vi "HiTechnic IRSeeker Sensor_AC all.vi"(0 "AC Mode":u8(ring) items=["1200 Hz", "600 Hz"], 2 "NXT":T4={"error"={"status"=FALSE, "code"=0, "source"=""}, "address"="", "NXT #"=-1, "Show Error"=TRUE, "Connection"=4} {"Connection" items=["USB", "Bluetooth", "USB then Bluetooth", "Last Connection", "Preference"]}, 3 "Port/MUX":T2 {"Port" items=["Port 1", "Port 2", "Port 3", "Port 4"]; "MUX Port" items=["No MUX", "MUX 1", "MUX 2", "MUX 3", "MUX 4"]}) -> (1 "All Info":T1, 4 "NXT":T4={"error"={"status"=FALSE, "code"=0, "source"=""}, "address"="", "NXT #"=-1, "Show Error"=TRUE, "Connection"=4} {"Connection" items=["USB", "Bluetooth", "USB then Bluetooth", "Last Connection", "Preference"]})   [LabVIEW 2009]
doc: "Reads the HiTechnic IRSeeker V2 Sensor in AC mode connected to the specified port and outputs a cluster containing the direction value as well an array of signal strengths from the five internal IR sensor elements. The direction value is in the range of 0 to 9 with 0 representing no IR detected; 1 to 9 represents a direction in a CW semi-circle around the sensor of which 5 indicates the IR source is straight ahead. In AC mode the sensor concentrates on a pulsating signal of either 600Hz or 1200Hz depending on the AC Mode setting.\n\n<B>Inputs\nNXT </B> connects to NXT terminal of previous VI to establish the flow of the program.\n<B>Port/MUX </B> is the port used for the sensor. This is a cluster that consists of the NXT port as well as the HiTechnic Sensor Multiplexer (MUX) port. If the MUX is not used, then set this field to <B>No MUX</B>.\n<B>AC Mode </B> can be set to either 600 Hz or 1200 Hz (default).\n\n<B>Outputs\nNXT </B> wires to NXT terminal of next VI to establish the flow of the program.\n<B>All Info </B> is a cluster containing the direction value as well as a 5 element array of signal strengths."
uses:
  <vilib>/NXT/Subs/LVHSConnector.ctl
  <vilib>/NXT/HiTechnic/subVIs/HiTechnic Port.ctl
  <vilib>/NXT/Block Support/NXT_InputPort.ctl
panel:
  in  "Previous Mode":u8[](array[ring])=[0, 0, 0, 0] items=["1200 Hz", "600 Hz"]
  # "HiTechnic IRSeeker Sensor VI\n\nThis VI reads the HiTechnic IRSeeker Sensor and \nreturns the current heading.\n\nFor more information go to www.hitechnic.com\nor email support@hitechnic.com\n(c) 2007 - 2009 HiTechnic"
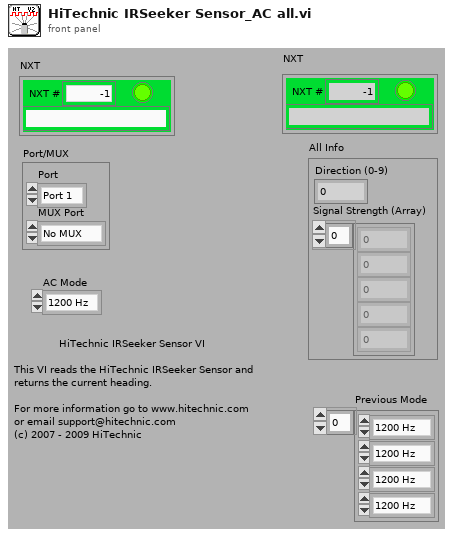
[diagram p1: front panel]
types:
  T1 = cluster{"Direction (0-9)":u8, "Signal Strength (Array)":u8[]}
  T2 = typedef "HiTechnic Port.ctl" = cluster{"Port":T3, "MUX Port":u8}
  T3 = typedef "NXT_InputPort.ctl" = u8
  T4 = typedef "LVHSConnector.ctl" = cluster{"error":errorcluster, "address":string, "NXT #":i32, "Show Error":bool, "Connection":u16}
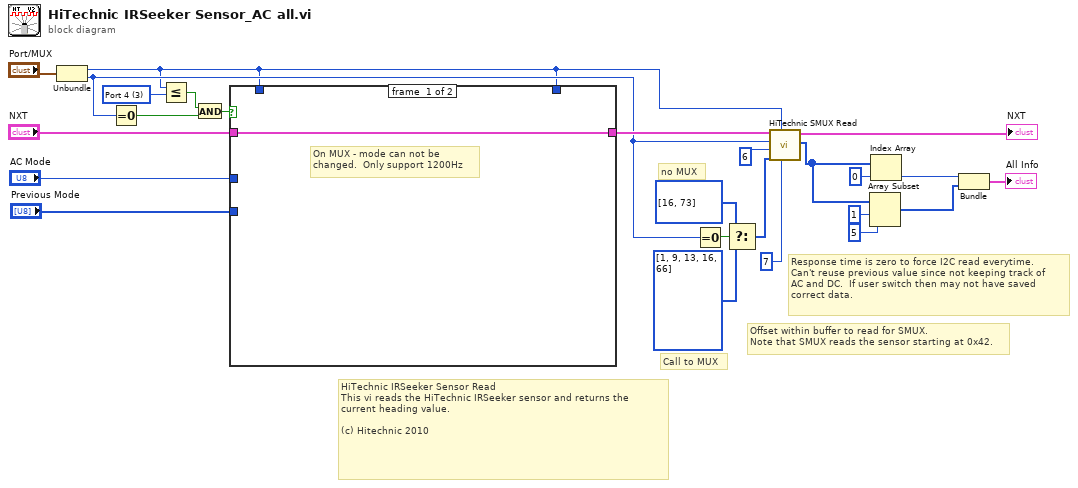
[diagram p0: block diagram]
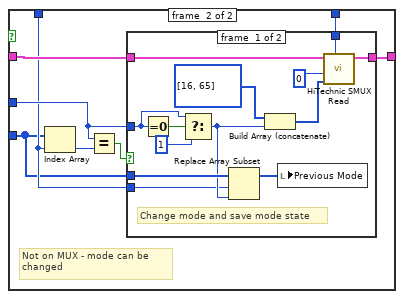
[diagram p2: hidden frame]
diagram:
  w4 = T3 3 items=["Port 1", "Port 2", "Port 3", "Port 4"] ("y")
  # "Response time is zero to force I2C read everytime.\nCan't reuse previous value since not keeping track of\nAC and DC.  If user switch then may not have saved \ncorrect data."
  # "Offset within buffer to read for SMUX.  \nNote that SMUX reads the sensor starting at 0x42."
  # "no MUX"
  # "Call to MUX"
  # "HiTechnic IRSeeker Sensor Read\nThis vi reads the HiTechnic IRSeeker sensor and returns the\ncurrent heading value.  \n\n(c) Hitechnic 2010"
  n1 = Unbundle("Port/MUX") -> ("Port"=w5:T3, "MUX Port"=w6:u8)
  n2 = Equal To 0?(x=w6) -> (x = 0?=w2:bool)
  n3 = Less Or Equal?(x=w5, y=w4) -> (x <= y?=w3:bool)
  n4 = And(x=w3, y=w2) -> (x .and. y?=w1:bool)
  n5 = case shown="True" w1 {
    tunnel: "NXT" -> [w26 w33]
    tunnel: [w26 w32] -> w9
    tunnel: "Previous Mode" -> [_ w28]
    tunnel: w5 -> [_ w30]
    tunnel: "AC Mode" -> [_ w31]
    tunnel: w5 -> [_ w29]
    frame #0 {
      # "On MUX - mode can not be\nchanged.  Only support 1200Hz"
    }
    frame #1 {
      # "Not on MUX - mode can be \nchanged"
      n6 = Index Array(array=w28, index=w30) -> (element=w34:u8)
      n7 = Equal?(x=w31, y=w34) -> (x = y?=w27:bool)
      n8 = case shown="True" w27 {
        tunnel: w33 -> [w46 w48]
        tunnel: [w45 w48] -> w32
        tunnel: w31 -> [w43 _]
        tunnel: w28 -> [w39 _]
        tunnel: w30 -> [w37 _]
        tunnel: w29 -> [w35 _]
        frame #0 {
          # "Change mode and save mode state"
          n9 = Equal To 0?(x=w43) -> (x = 0?=w44:bool)
          n10 = Select(t=w43, s=w44, f=u8 1) -> (s? t:f=w38:u8)
          n11 = Replace Array Subset(array=w39, new element=w38, index=w37) -> (w36:u8[])
          n12 = Build Array (concatenate)(u8[] [16, 65] ("Buffer"), w38) -> (w40:u8[])
          n13 = local write "Previous Mode"(w36) -> ()
          n14 = call <vilib>:"HiTechnic SMUX Read.vi"("Port"=w35, "Parameters"=w40, "Read Length"=0, "NXT"=w46) -> ("NXT"=w45:T4)  [unwired: 6 in, 1 out]
        }
        frame #1 {
          # "Mode not changed."
        }
      }
    }
  }
  n15 = Equal To 0?(x=w6) -> (x = 0?=w22:bool)
  n16 = Select(t=u8[] [16, 73] ("Buffer"), s=w22, f=u8[] [1, 9, 13, 16, 66]) -> (s? t:f=w25:u8[])
  n17 = call <vilib>:"HiTechnic SMUX Read.vi"("Offset"=u8 7, "Port"=w5, "Parameters"=w25, "Read Length"=u8 6, "MUX Port"=w6, "NXT"=w9) -> ("Array"=w12:u8[], "NXT"=→"NXT":T4)  [unwired: 4 in]
  n18 = Array Subset(array=w12, index=1, length=5) -> (w13:u8[])
  n19 = Index Array(array=w12, index=0) -> (element=w17:u8)
  n20 = Bundle("Numeric"=w17, w13) -> (→"All Info":cluster{"Numeric":u8, u8[]})  [unwired: 1 in]
